vi "Measurement Logic.vi"() -> ()   [LabVIEW 2021, in "Voltage Measurement.lvlib"]
uses:
  Voltage Measurement.lvlib
  <vilib>/Plug-In SDKs/Measurements/Measure Call Context/Measure Call Context.lvclass
  <vilib>/Plug-In SDKs/Sessions/niDMM/NI Session Management niDMM.lvlib
  <vilib>/Plug-In SDKs/Sessions/niDCPower/NI Session Management niDCPower.lvlib
  <vilib>/Plug-In SDKs/Clients/Session Management V1/Session Reservation/Session Reservation.lvclass
  ec50b443-56b4-4650-b870-3e73b6de3c7c.vi
  d11d6585-437b-4326-b166-854f3e8d2707.vi
  Measurement Configuration.ctl
  Measurement Results.ctl
  <instrlib>/niDMM/nidmm.llb/niDMM Resolution in Digits.ctl
panel:
  out "measure call context out":refnum<class "Measure Call Context.lvclass">
  in  "measure call context in":refnum<class "Measure Call Context.lvclass">
  out "measurement results":T1={"Measurement "=0.0, "Signal Out of Range"=FALSE, "Measurement from SMU Str"="Empty", "Waveform Graph"=[0.0]} {"Measurement" format="%.6p"}
  in  "measurement configuration":T2={"Vin SMU Channel"="Lorem ipsum dolor sit", "Range"=1.2, "Resolution in Digits"=0.0, "Voltage Config Str"="", "Current Config Str"="", "Vin SMU Pin"="", "Device Name Pin"=""} {"Resolution in Digits" items=["3 1/2"=3.5, "4 1/2"=4.5, "5 1/2"=5.5, "6 1/2"=6.5, "7 1/2"=7.5]}
  out "error out":errorcluster
  in  "error in":errorcluster
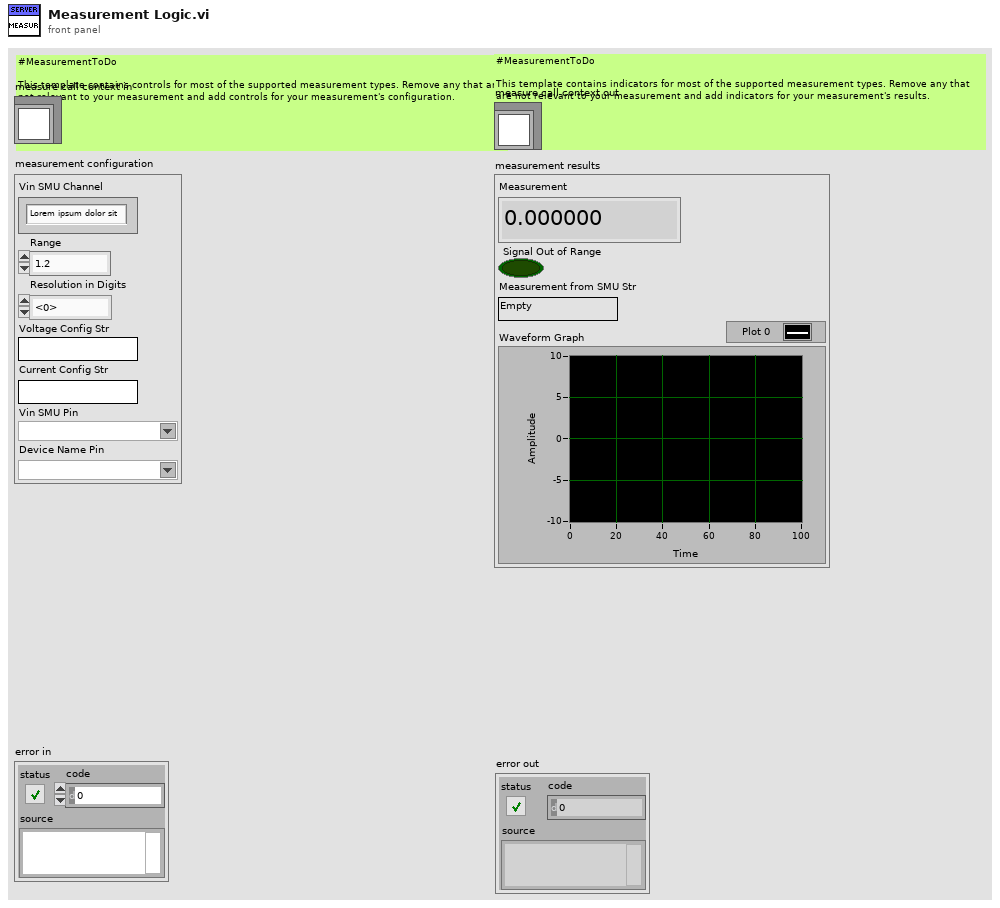
[diagram p1: front panel]
types:
  T1 = typedef "Voltage Measurement.lvlib/Measurement Results.ctl" = cluster{"Measurement ":dbl, "Signal Out of Range":bool, "Measurement from SMU Str":string, "Waveform Graph":dbl[]}
  T2 = typedef "Voltage Measurement.lvlib/Measurement Configuration.ctl" = cluster{"Vin SMU Channel":string, "Range":dbl, "Resolution in Digits":T3, "Voltage Config Str":string, "Current Config Str":string, "Vin SMU Pin":string, "Device Name Pin":string}
  T3 = typedef "niDMM Resolution in Digits.ctl" = dbl
  T4 = typedef "NI Session Management niDMM.lvlib/Connection with Session.ctl" = cluster{"connection":T5, "session":refnum<k15>}
  T5 = typedef "NI Session Management V1 Client.lvlib/Session Reservation.lvclass/Connection.ctl" = cluster{"pin or relay name":string, "site":i32, "instrument type id":string, "channel":string}
  T6 = typedef "NI Session Management niDCPower.lvlib/Connection with Session.ctl" = cluster{"connection":T5, "session":refnum<k15>}
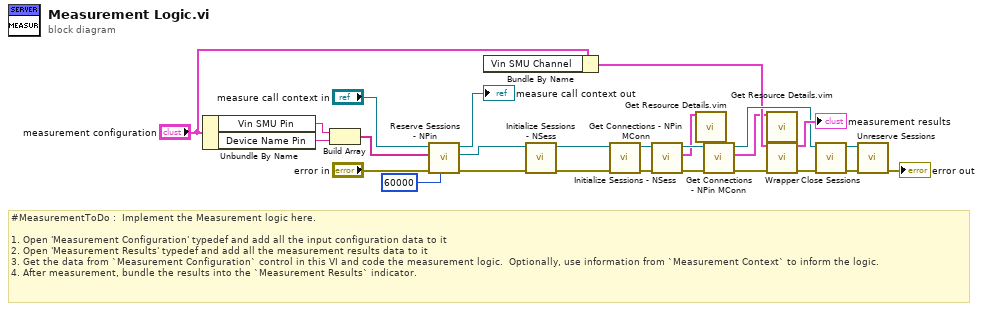
[diagram p0: block diagram]
diagram:
  # "#MeasurementToDo :  Implement the Measurement logic here.\n\n1. Open 'Measurement Configuration' typedef and add all the input configuration data to it\n2. Open 'Measurement Results' typedef and add all the measurement results data to it\n3. Get the data from `Measurement Configuration` control in this VI and code the measurement logic.  Optionally, use information from `Measurement Context` to inform the logic.\n4. After measurement, bundle the results into the `Measurement Results` indicator."
  n1 = Unbundle By Name("measurement configuration") -> ("Vin SMU Pin"=w25:string, "Device Name Pin"=w24:string)
  n2 = Build Array(w25, w24) -> (w20:string[])
  n3 = call <vilib>:"Reserve Sessions - NPin.vi"("timeout (ms)"=60000, "error in"="error in", "pin or relay names"=w20, "measurement context in"="measure call context in") -> ("error out"=w18:errorcluster, "session reservation out"=w17:refnum<class "Session Reservation.lvclass">, "measurement context out"=→"measure call context out":refnum<class "Measure Call Context.lvclass">)  [unwired: 5 in]
  n4 = Bundle By Name(cluster="measurement configuration") -> (w2:T2)  [unwired: 1 in]
  n5 = call <vilib>:"Initialize Sessions - NSess.vi"("error in"=w18, "session reservation in"=w17) -> ("error out"=w16:errorcluster, "session reservation out"=w15:refnum<class "Session Reservation.lvclass">)  [unwired: 6 in, 2 out]
  n6 = call <vilib>:"Initialize Sessions - NSess.vi"("error in"=w16, "session reservation in"=w15) -> ("error out"=w14:errorcluster, "session reservation out"=w13:refnum<class "Session Reservation.lvclass">)  [unwired: 6 in, 2 out]
  n7 = call <vilib>:"Get Connections - NPin MConn.vi"("error in"=w14, "session reservation in"=w13) -> ("error out"=w12:errorcluster, "connections"=w3:T4[], "session reservation out"=w11:refnum<class "Session Reservation.lvclass">)  [unwired: 7 in]
  n8 = call "Get Resource Details.vim"("connections"=w3) -> ()  [unwired: 13 in, 2 out]
  n9 = call <vilib>:"Get Connections - NPin MConn.vi"("error in"=w12, "session reservation in"=w11) -> ("error out"=w9:errorcluster, "connections"=w1:T6[], "session reservation out"=w7:refnum<class "Session Reservation.lvclass">)  [unwired: 7 in]
  n10 = call "Get Resource Details.vim"("connections"=w1) -> ()  [unwired: 13 in, 2 out]
  n11 = call "Wrapper.vi"("measurement configuration"=w2, "error in"=w9) -> ("measurement results"=→"measurement results":T1, "error out"=w8:errorcluster)  [unwired: 12 in]
  n12 = call <vilib>:"Close Sessions.vi"("error in"=w8, "session reservation in"=w7) -> ("error out"=w5:errorcluster, "session reservation out"=w4:refnum<class "Session Reservation.lvclass">)  [unwired: 8 in]
  n13 = call <vilib>:"Unreserve Sessions.vi"("error in"=w5, "session reservation in"=w4) -> ("error out"=→"error out":errorcluster)  [unwired: 9 in]
